vi "Angle_4_R4.vi"() -> ()   [LabVIEW 2020]
uses:
  Support/Controls/Clst_Initialize Input.ctl
  Support/Controls/Cmd_Var Data IO.ctl
  Support/Controls/Cmd_Mouse Popup.ctl
  Variables/Global_Cal Info.vi
panel:
  out "최소범위":string
  in  "표시방식":string(combo)
  out "단위":string
  out "최대범위":string
  in  "Spec 변경":bool
  in  "Random":bool
  out "Resolution":string[][](table) caption="Spec"
  out "Spec":string[][](table)
  out "제목":string
  out "에러 출력":errorcluster
  out "Condition":string[][](table) caption="2. 직선성 시험"
  in  "최소눈금":string(combo)
  in  "Measured":string[][](table)
  out "Load?":bool
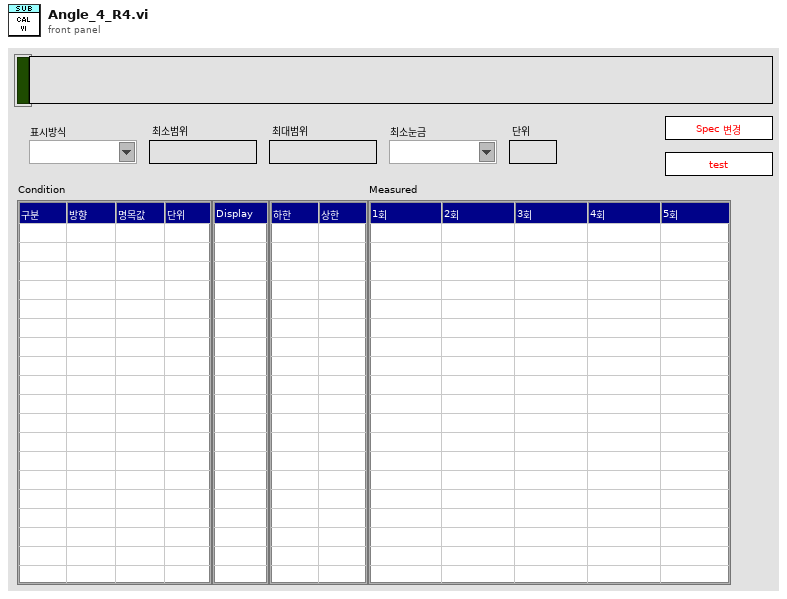
[diagram p1: front panel]
types:
  T1 = typedef "Cmd_Mouse Popup.ctl" = enum16{"활성화", "메뉴선택"}
  T2 = cluster{"Shift":bool, "Ctrl":bool, "Alt":bool, "Cmd":bool, "Opt":bool}
  T3 = typedef "Clst_Initialize Input.ctl" = cluster{"Initialize 1":cluster{"Condition":refnum<vi>[], "Spec":refnum<vi>[], "Measured":refnum<vi>[], "Resolution":refnum<vi>[], "Func_ext":string, "제목":refnum<vi>, "Measured_ADJ":refnum<vi>[]}, "Initialize 2":cluster{"문자열":refnum<vi>[], "콤보박스":refnum<vi>[], "링":refnum<vi>[], "열거형":refnum<vi>[], "테이블":refnum<vi>[], "여러열":refnum<vi>[], "디지털(DBL)":refnum<vi>[], "3D string":refnum<vi>[], "ctrl":refnum<vi>[], "boolean":refnum<vi>[]}}
  T4 = typedef "Cmd_Var Data IO.ctl" = enum16{"Condition", "Condition Default", "Condition_Temp", "Resolution", "Resolution Default", "Resolution Old", "Spec", "Spec Default", "Spec Old", "Spec Temp", "Result", "Result2", "Result3", "Result_Temp", "Result_ADJ", "Result_ADJ2", "STD1", "STD2", "STD3", "STD4", "STD5", "STD Temp", "CMC", "CMC Default"}
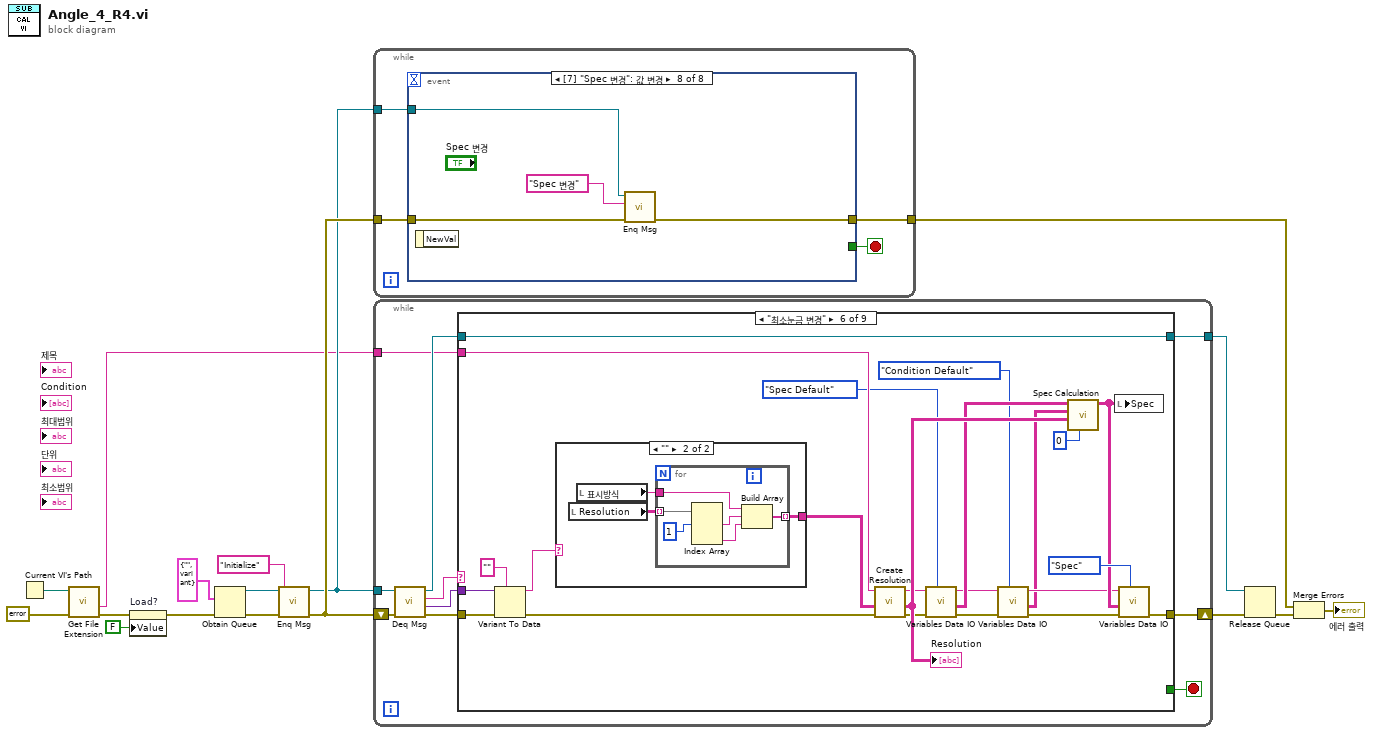
[diagram p0: block diagram]
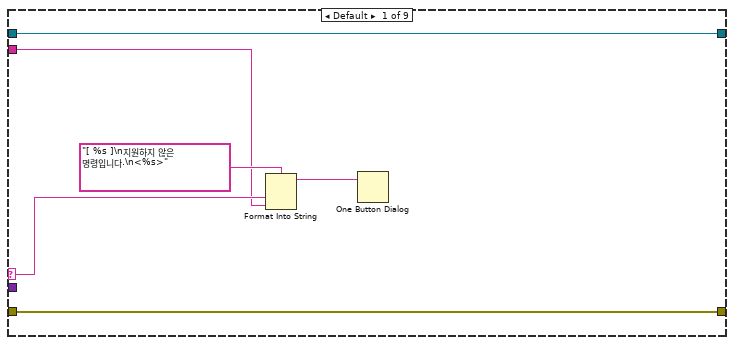
[diagram p2: hidden frame]
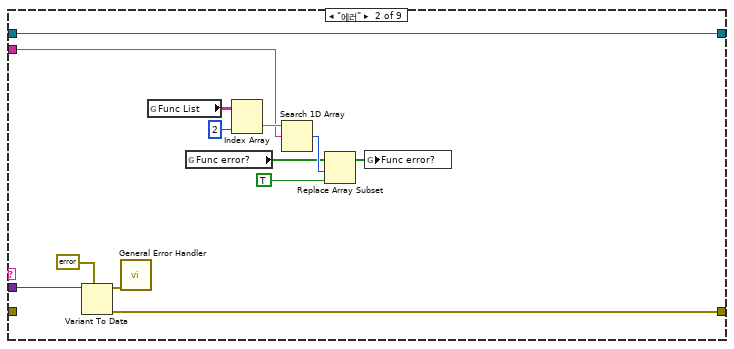
[diagram p3: hidden frame]
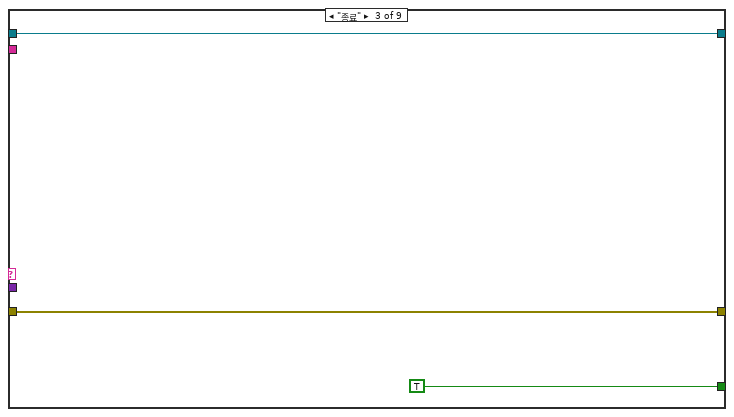
[diagram p4: hidden frame]
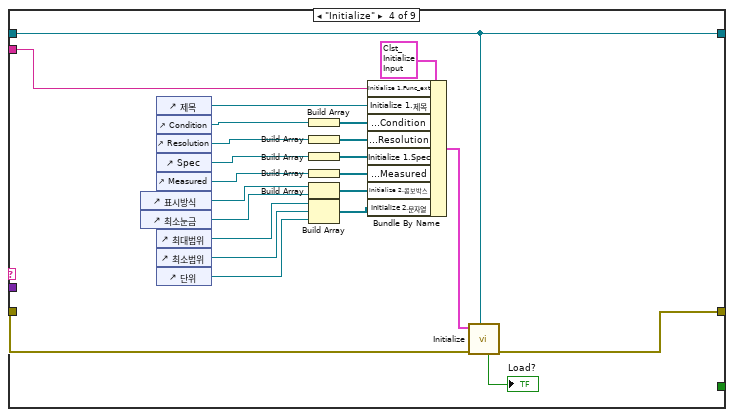
[diagram p5: hidden frame]
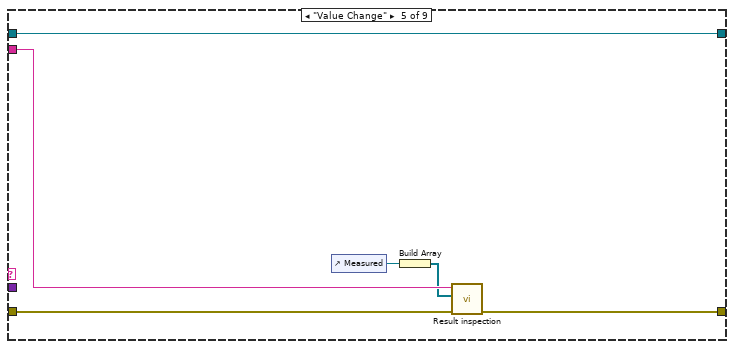
[diagram p6: hidden frame]
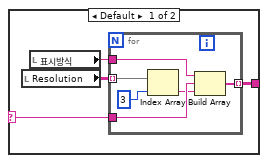
[diagram p7: hidden frame]
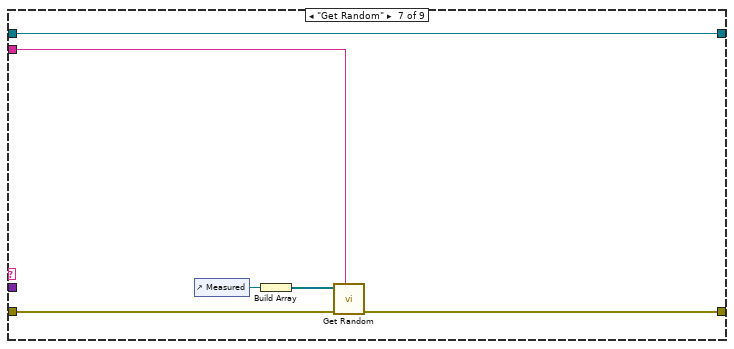
[diagram p8: hidden frame]
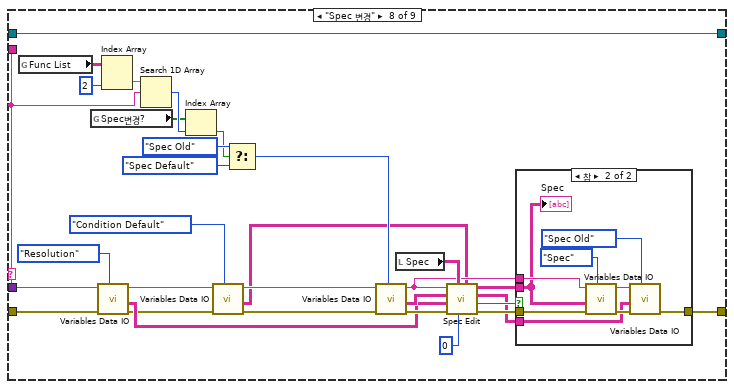
[diagram p9: hidden frame]
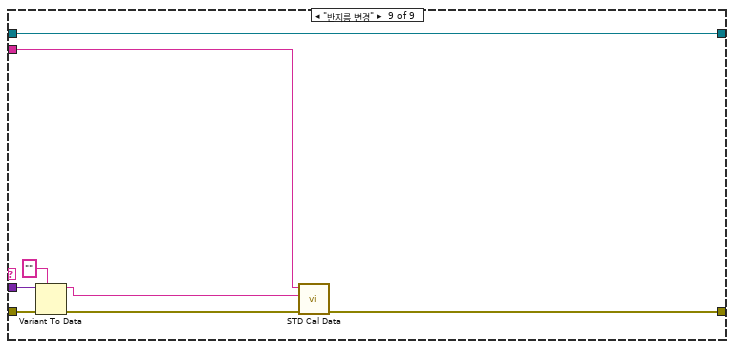
[diagram p11: hidden frame]
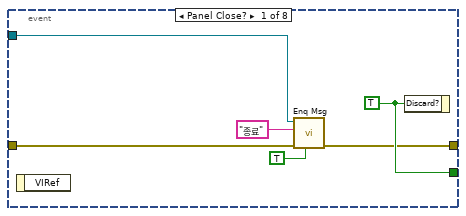
[diagram p12: hidden frame]
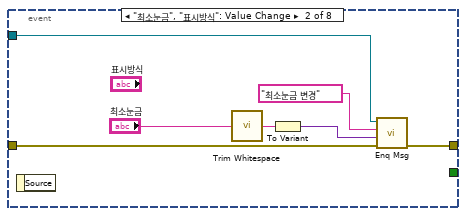
[diagram p13: hidden frame]
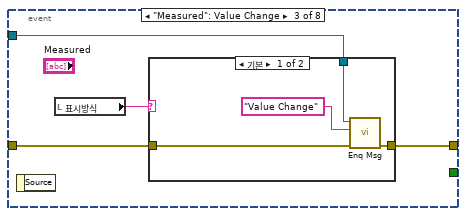
[diagram p14: hidden frame]
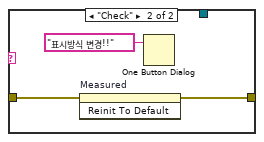
[diagram p15: hidden frame]
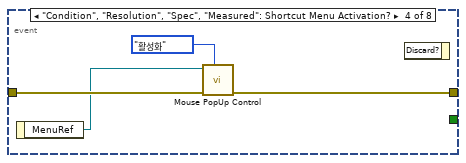
[diagram p16: hidden frame]
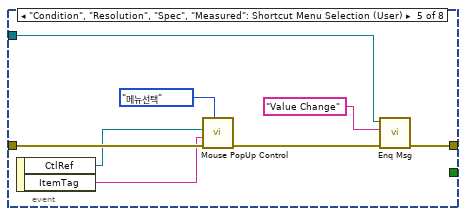
[diagram p17: hidden frame]
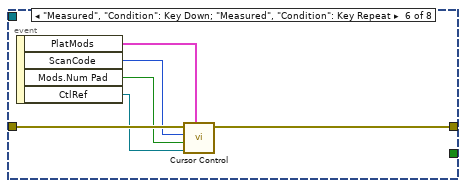
[diagram p18: hidden frame]
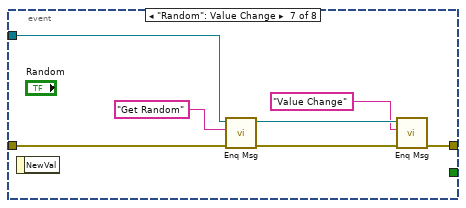
[diagram p19: hidden frame]
diagram:
  n1 = Current VI's Path() -> (path=w5:path)
  n2 = call <vilib>:"Get File Extension.vi"("error in (no error)"=errorcluster {"status"=FALSE, "code"=0, "source"=""} ("에러 상수"), "file"=w5) -> ("error out"=w3:errorcluster, "filename without extension"=w4:string)  [unwired: 5 in, 3 out]
  n3 = property on="Load?" class="Bool (엄격한)"(error in=w3, "Value"=FALSE ("Load?")) -> (error out=w2:errorcluster)  [unwired: 1 in, 1 out]
  n4 = Obtain Queue(element data type=cluster{"메세지":string, "값":variant} {"메세지"="", "값"=variant} ("Message Cluster"), error in (no error)=w2) -> (queue out=w14:refnum<queue>, error out=w16:errorcluster)  [unwired: 3 in, 1 out]
  n5 = call "Enq Msg.vi"("에러 입력(에러 없음)"=w16, "메세지"="Initialize", "큐 입력"=w14) -> ("에러 출력"=w15:errorcluster, "큐 출력"=w12:refnum<queue>)  [unwired: 7 in]
  n6 = while {
    tunnel: w15 -> [w19]
    tunnel: w12 -> [w20]
    tunnel: [w18] -> w9
    stop <- w21 stop-if-true
    n7 = event shown="[7] \"Spec 변경\": 값 변경" {
      selector: _ -> [_ _ _ _ _ _ _ _]
      dyn-events: _ -> [_ _ _ _ _ _ _ _]
      timeout: _ -> [_ _ _ _ _ _ _ _]
      tunnel: [w27 _ _ _ _ _ _ _] -> w21
      tunnel: w20 -> [w25 w33 w38 _ w50 _ w68 w72]
      tunnel: w19 -> [w26 w34 w36 w49 w57 w63 w69 w73]
      tunnel: [w23 w32 w37 w48 w51 w62 w64 w71] -> w18
      event Panel Close? {
        w27 = TRUE ("버림?")
        n8 = event-data() -> ()  [unwired: 1 in, 1 out]
        n9 = call "Enq Msg.vi"("우선순위 메시지?"=TRUE, "에러 입력(에러 없음)"=w26, "메세지"="종료", "큐 입력"=w25) -> ("에러 출력"=w23:errorcluster)  [unwired: 6 in, 1 out]
        n10 = event-data("Discard?"=w27) -> ()  [unwired: 1 in, 1 out]
      }
      event "최소눈금", "표시방식": Value Change {
        n11 = event-data() -> ()  [unwired: 1 in, 1 out]
        n12 = call <vilib>:"Trim Whitespace.vi"("string"="최소눈금") -> ("trimmed string"=w30:string)  [unwired: 1 in]
        n13 = To Variant(anything=w30) -> (Variant=w28:variant)
        n14 = call "Enq Msg.vi"("에러 입력(에러 없음)"=w34, "값"=w28, "메세지"="최소눈금 변경", "큐 입력"=w33) -> ("에러 출력"=w32:errorcluster)  [unwired: 6 in, 1 out]
      }
      event "Measured": Value Change {
        n15 = event-data() -> ()  [unwired: 1 in, 1 out]
        n16 = local read "표시방식"() -> (w35:string)
        n17 = case shown="기본" w35 {
          tunnel: w38 -> [w42 _]
          tunnel: [w41 w43] -> w37
          tunnel: w36 -> [w40 w44]
          frame Default {
            n18 = call "Enq Msg.vi"("에러 입력(에러 없음)"=w40, "메세지"="Value Change", "큐 입력"=w42) -> ("에러 출력"=w41:errorcluster)  [unwired: 7 in, 1 out]
          }
          frame "Check" {
            n19 = invoke on="Measured" class="Tbl (엄격한)" method="Reinit To Default"(error in=w44) -> (error out=w43:errorcluster)  [unwired: 2 in, 2 out]
            n20 = One Button Dialog(message="표시방식 변경!!" ("메시지")) -> ()  [unwired: 1 in, 1 out]
          }
        }
      }
      event "Condition", "Resolution", "Spec", "Measured": Shortcut Menu Activation? {
        n21 = event-data() -> ("MenuRef"=w47:refnum<k9>)  [unwired: 1 in]
        n22 = call "Mouse PopUp Control.vi"("type"=Cmd_Mouse_Popup."활성화", "error in"=w49, "메뉴 참조"=w47) -> ("error out"=w48:errorcluster)  [unwired: 8 in]
        n23 = event-data() -> ()  [unwired: 2 in, 1 out]
      }
      event "Condition", "Resolution", "Spec", "Measured": Shortcut Menu Selection (User) {
        n24 = event-data() -> ("CtlRef"=w55:refnum<vi>, "ItemTag"=w54:string)  [unwired: 1 in]
        n25 = call "Mouse PopUp Control.vi"("type"=Cmd_Mouse_Popup."메뉴선택", "error in"=w57, "아이템 태그"=w54, "Tbl 참조 번호"=w55) -> ("error out"=w52:errorcluster)  [unwired: 7 in]
        n26 = call "Enq Msg.vi"("에러 입력(에러 없음)"=w52, "메세지"="Value Change", "큐 입력"=w50) -> ("에러 출력"=w51:errorcluster)  [unwired: 7 in, 1 out]
      }
      event "Measured", "Condition": Key Down; "Measured", "Condition": Key Repeat {
        n27 = event-data() -> ("PlatMods"=w58:T2, "ScanCode"=w61:i16, "Mods.Num Pad"=w60:bool, "CtlRef"=w59:refnum<vi>)  [unwired: 1 in]
        n28 = call "Cursor Control.vi"("플랫폼 조합키"=w58, "참조"=w59, "Num Pad"=w60, "ScanCode"=w61, "error in"=w63) -> ("error out"=w62:errorcluster)  [unwired: 5 in, 1 out]
      }
      event "Random": Value Change {
        n29 = event-data() -> ()  [unwired: 1 in, 1 out]
        n30 = call "Enq Msg.vi"("에러 입력(에러 없음)"=w69, "메세지"="Get Random", "큐 입력"=w68) -> ("에러 출력"=w67:errorcluster, "큐 출력"=w66:refnum<queue>)  [unwired: 7 in]
        n31 = call "Enq Msg.vi"("에러 입력(에러 없음)"=w67, "메세지"="Value Change", "큐 입력"=w66) -> ("에러 출력"=w64:errorcluster)  [unwired: 7 in, 1 out]
      }
      event "Spec 변경": Value Change {
        n32 = event-data() -> ()  [unwired: 1 in, 1 out]
        n33 = call "Enq Msg.vi"("에러 입력(에러 없음)"=w73, "메세지"="Spec 변경", "큐 입력"=w72) -> ("에러 출력"=w71:errorcluster)  [unwired: 7 in, 1 out]
      }
    }
  }
  n34 = while {
    shift-right: [w84] -> w11
    shift-left: w15 -> [w83]
    tunnel: w12 -> [w81]
    tunnel: [w76] -> w10
    tunnel: w4 -> [w75]
    stop <- w77 stop-if-true
    n35 = call "Deq Msg.vi"("에러 입력(에러 없음)"=w83, "큐 입력"=w81) -> ("에러 출력"=w82:errorcluster, "값"=w78:variant, "메세지"=w80:string, "큐 출력"=w79:refnum<queue>)  [unwired: 6 in]
    n36 = case shown="\"최소눈금 변경\"" w80 {
      selector: w80 -> [w86 _ _ _ _ _ _ _ _]
      tunnel: w82 -> [w90 _ w106 w129 w132 w157 w179 w206 w230]
      tunnel: [w90 w100 w106 w109 w134 w150 w180 w209 w224] -> w84
      tunnel: w79 -> [w89 w99 w104 w114 w135 w158 w183 w213 w231]
      tunnel: w78 -> [_ w101 _ _ _ w156 _ _ w228]
      tunnel: [_ _ TRUE ("버림?") _ _ _ _ _ _] -> w77
      tunnel: [w89 w99 w104 w114 w135 w158 w183 w213 w231] -> w76
      tunnel: w75 -> [w85 w91 _ w115 w133 w154 w178 w192 w225]
      frame Default {
        n37 = Format Into String(format string="[ %s ]\n지원하지 않은 명령입니다.\n<%s>" ("메시지"), w86, w85) -> (resulting string=w87:string)  [unwired: 2 in, 1 out]
        n38 = One Button Dialog(message=w87) -> ()  [unwired: 1 in, 1 out]
      }
      frame "에러" {
        n39 = Variant To Data(type=errorcluster {"status"=FALSE, "code"=0, "source"=""} ("에러 출력"), Variant=w101) -> (data=w103:errorcluster, error out=w100:errorcluster)  [unwired: 1 in]
        n40 = call <vilib>:"General Error Handler.vi"("error in (no error)"=w103) -> ()  [unwired: 10 in, 5 out]
        n41 = global read "Global_Cal Info.vi" "Func List"() -> (w93:string[][])
        n42 = global read "Global_Cal Info.vi" "Func error?"() -> (w96:bool[])
        n43 = Index Array(array=w93, index (col)=2 ("비활성화된 인덱스 (열)")) -> (element=w94:string[])  [unwired: 1 in]
        n44 = Search 1D Array(1D array=w94, element=w91) -> (index of element=w97:i32)  [unwired: 1 in]
        n45 = Replace Array Subset(array=w96, new element=TRUE ("새 원소/부분배열"), index=w97) -> (w98:bool[])
        n46 = global write "Global_Cal Info.vi" "Func error?"(w98) -> ()
      }
      frame "종료" {
      }
      frame "Initialize" {
        n47 = control-ref of="표시방식"() -> (w113:refnum<vi>)
        n48 = control-ref of="최소눈금"() -> (w122:refnum<vi>)
        n49 = control-ref of="제목"() -> (w120:refnum<vi>)
        n50 = control-ref of="Condition"() -> (w126:refnum<vi>)
        n51 = control-ref of="Resolution"() -> (w116:refnum<vi>)
        n52 = control-ref of="Spec"() -> (w119:refnum<vi>)
        n53 = control-ref of="Measured"() -> (w123:refnum<vi>)
        n54 = control-ref of="최대범위"() -> (w108:refnum<vi>)
        n55 = control-ref of="최소범위"() -> (w110:refnum<vi>)
        n56 = control-ref of="단위"() -> (w112:refnum<vi>)
        n57 = Build Array(w126) -> (w125:refnum<vi>[])
        n58 = Build Array(w116) -> (w117:refnum<vi>[])
        n59 = Build Array(w119) -> (w118:refnum<vi>[])
        n60 = Build Array(w123) -> (w124:refnum<vi>[])
        n61 = Build Array(w113, w122) -> (w121:refnum<vi>[])
        n62 = Build Array(w108, w110, w112) -> (w111:refnum<vi>[])
        n63 = Bundle By Name(cluster=T3 {"Initialize 1"={"Condition"=[], "Spec"=[], "Measured"=[], "Resolution"=[], "Func_ext"="", "제목"=refnum, "Measured_ADJ"=[]}, "Initialize 2"={"문자열"=[], "콤보박스"=[], "링"=[], "열거형"=[], "테이블"=[], "여러열"=[], "디지털(DBL)"=[], "3D string"=[], "ctrl"=[], "boolean"=[]}} ("입력 클러스터"), "Initialize 1.Func_ext"=w115, "Initialize 1.제목"=w120, "Initialize 1.Condition"=w125, "Initialize 1.Resolution"=w117, "Initialize 1.Spec"=w118, "Initialize 1.Measured"=w124, "Initialize 2.콤보박스"=w121, "Initialize 2.문자열"=w111) -> (w127:T3)
        n64 = call "Initialize.vi"("큐 입력"=w114, "error in"=w129, "입력 클러스터"=w127) -> ("error out"=w109:errorcluster, "Load?"=→"Load?":bool)  [unwired: 5 in, 2 out]
      }
      frame "Value Change" {
        n65 = control-ref of="Measured"() -> (w131:refnum<vi>)
        n66 = Build Array(w131) -> (w130:refnum<vi>[])
        n67 = call "Result inspection.vi"("error in"=w132, "Ref. Data (Inspection)"=w130, "Func ext"=w133) -> ("error out"=w134:errorcluster)  [unwired: 5 in, 3 out]
      }
      frame "최소눈금 변경" {
        n68 = Variant To Data(error in=w157, type="", Variant=w156) -> (data=w143:string, error out=w145:errorcluster)
        n69 = case shown="\"\"" w143 {
          selector: w143 -> [w159 _]
          tunnel: [w162 w171] -> w144
          frame Default {
            n70 = local read "Resolution"() -> (w161:string[][])
            n71 = local read "표시방식"() -> (w160:string)
            n72 = for {
              tunnel: w161 -> [w168] mode=indexing
              tunnel: w159 -> [w167]
              tunnel: [w165] -> w162 mode=indexing
              tunnel: w160 -> [w164]
              n73 = Index Array(array=w168, index=3 ("인덱스")) -> (element=w166:string)
              n74 = Build Array(w164, w167, w166) -> (w165:string[])
            }
          }
          frame "" {
            n75 = local read "Resolution"() -> (w170:string[][])
            n76 = local read "표시방식"() -> (w169:string)
            n77 = for {
              tunnel: w170 -> [w177] mode=indexing
              tunnel: [w176] -> w171 mode=indexing
              tunnel: w169 -> [w175]
              n78 = Index Array(array=w177, index #1=1 ("인덱스")) -> (element #1=w173:string, element #3=w172:string)  [unwired: 2 in, 1 out]
              n79 = Build Array(w175, w173, w172) -> (w176:string[])
            }
          }
        }
        n80 = call "Create Resolution.vi"("에러 입력(에러 없음)"=w145, "Resolution"=w144, "Func_ext"=w154) -> ("에러 출력"=w148:errorcluster, "Resolution Out"=w151:string[][], "Func_ext 출력"=w147:string)  [unwired: 6 in]
        "Resolution" <- w151
        n81 = call "Variables Data IO.vi"("Select"=Cmd_Var_Data_IO."Spec Default", "error in"=w148, "Func_ext"=w147) -> ("error out"=w139:errorcluster, "Data Out"=w146:string[][], "Func_ext Out"=w140:string)  [unwired: 6 in]
        n82 = call "Variables Data IO.vi"("Select"=Cmd_Var_Data_IO."Condition Default", "error in"=w139, "Func_ext"=w140) -> ("error out"=w137:errorcluster, "Data Out"=w136:string[][], "Func_ext Out"=w138:string)  [unwired: 6 in]
        n83 = call "Spec Calculation.vi"("기준값 열번호"=0 ("열번호(기준값)"), "Resolution"=w151, "Condition in"=w136, "Spec Default"=w146) -> ("Spec out"=w142:string[][])  [unwired: 6 in, 1 out]
        n84 = local write "Spec"(w142) -> ()
        n85 = call "Variables Data IO.vi"("Select"=Cmd_Var_Data_IO."Spec", "error in"=w137, "Data In"=w142, "Func_ext"=w138) -> ("error out"=w150:errorcluster)  [unwired: 5 in, 2 out]
      }
      frame "Get Random" {
        n86 = control-ref of="Measured"() -> (w182:refnum<vi>)
        n87 = Build Array(w182) -> (w181:refnum<vi>[])
        n88 = call "Get Random.vi"("Func_Ext"=w178, "에러 입력"=w179, "Meas"=w181) -> ("에러 출력"=w180:errorcluster)  [unwired: 7 in, 1 out]
      }
      frame "Spec 변경" {
        n89 = global read "Global_Cal Info.vi" "Func List"() -> (w197:string[][])
        n90 = global read "Global_Cal Info.vi" "Spec변경?"() -> (w193:bool[])
        n91 = call "Variables Data IO.vi"("Select"=Cmd_Var_Data_IO."Resolution", "error in"=w206, "Func_ext"=w192) -> ("error out"=w188:errorcluster, "Data Out"=w190:string[][], "Func_ext Out"=w189:string)  [unwired: 6 in]
        n92 = Index Array(array=w197, index (col)=2 ("비활성화된 인덱스 (열)")) -> (element=w195:string[])  [unwired: 1 in]
        n93 = Search 1D Array(1D array=w195, element=w192) -> (index of element=w194:i32)  [unwired: 1 in]
        n94 = Index Array(array=w193, index=w194) -> (element=w198:bool)
        n95 = call "Variables Data IO.vi"("Select"=Cmd_Var_Data_IO."Condition Default", "error in"=w188, "Func_ext"=w189) -> ("error out"=w187:errorcluster, "Data Out"=w184:string[][], "Func_ext Out"=w186:string)  [unwired: 6 in]
        n96 = Select(t=Cmd_Var_Data_IO."Spec Old" ("Select"), s=w198, f=Cmd_Var_Data_IO."Spec Default" ("Select")) -> (s? t:f=w191:T4)
        n97 = call "Variables Data IO.vi"("Select"=w191, "error in"=w187, "Func_ext"=w186) -> ("error out"=w208:errorcluster, "Data Out"=w201:string[][], "Func_ext Out"=w202:string)  [unwired: 6 in]
        n98 = local read "Spec"() -> (w203:string[][])
        n99 = call "Spec Edit.vi"("Condition"=w184, "열번호(기준값)"=0, "Spec Value"=w203, "에러 입력(에러 없음)"=w208, "Resolution"=w190, "Spec Default"=w201, "Func_ext"=w202) -> ("에러 출력"=w210:errorcluster, "변경?"=w211:bool, "Spec Default out"=w205:string[][], "Spec 출력"=w212:string[][])  [unwired: 1 in]
        n100 = case shown="참" w211 {
          tunnel: w212 -> [_ w220]
          tunnel: w210 -> [w214 w223]
          tunnel: [w214 w218] -> w209
          tunnel: w202 -> [_ w221]
          tunnel: w205 -> [_ w216]
          frame False {
          }
          frame True {
            n101 = call "Variables Data IO.vi"("Select"=Cmd_Var_Data_IO."Spec", "error in"=w223, "Data In"=w220, "Func_ext"=w221) -> ("error out"=w219:errorcluster, "Func_ext Out"=w217:string)  [unwired: 5 in, 1 out]
            n102 = call "Variables Data IO.vi"("Select"=Cmd_Var_Data_IO."Spec Old", "error in"=w219, "Data In"=w216, "Func_ext"=w217) -> ("error out"=w218:errorcluster)  [unwired: 5 in, 2 out]
            "Spec" <- w220
          }
        }
      }
      frame "반지름 변경" {
        n103 = Variant To Data(error in=w230, type="", Variant=w228) -> (data=w226:string, error out=w229:errorcluster)
        n104 = call "STD Cal Data.vi"("error in"=w229, "문자열"=w226, "Func_ext"=w225) -> ("error out"=w224:errorcluster)  [unwired: 4 in, 4 out]
      }
    }
  }
  n105 = Release Queue(queue=w10, error in (no error)=w11) -> (error out=w8:errorcluster)  [unwired: 1 in, 2 out]
  n106 = Merge Errors(w9, w8) -> (→"에러 출력":errorcluster)
